vi "4Pi Capture Scan Counter.vi"(8 "Scan Tracker":T1) -> (0 "Scan Tracker Out":T1, 1 "Move stage?":bool, 2 "F_MVR/T_MOV":bool, 3 "Exit?":bool)   [LabVIEW 2021]
uses:
  4Pi Capture Manager Controls/4Pi Capture Scan Tracker.ctl
  4Pi Capture Manager Controls/4Pi Capture Switch Laser.ctl
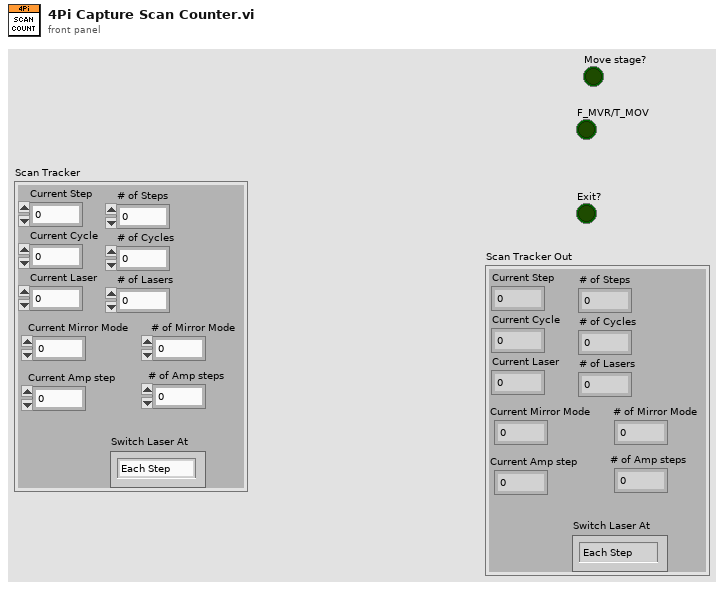
[diagram p1: front panel]
types:
  T1 = typedef "4Pi Capture Scan Tracker.ctl" = cluster{"Current Step":u16, "Current Cycle":u16, "Current Laser":u16, "# of Lasers":u16, "# of Cycles":u16, "# of Steps":u16, "Switch Laser At":T2, "Current Mirror Mode":u16, "# of Mirror Mode":u16, "Current Amp step":u16, "# of Amp steps":u16}
  T2 = typedef "4Pi Capture Switch Laser.ctl" = enum16{"Each Step", "Each Cycle", "All Cycles"}
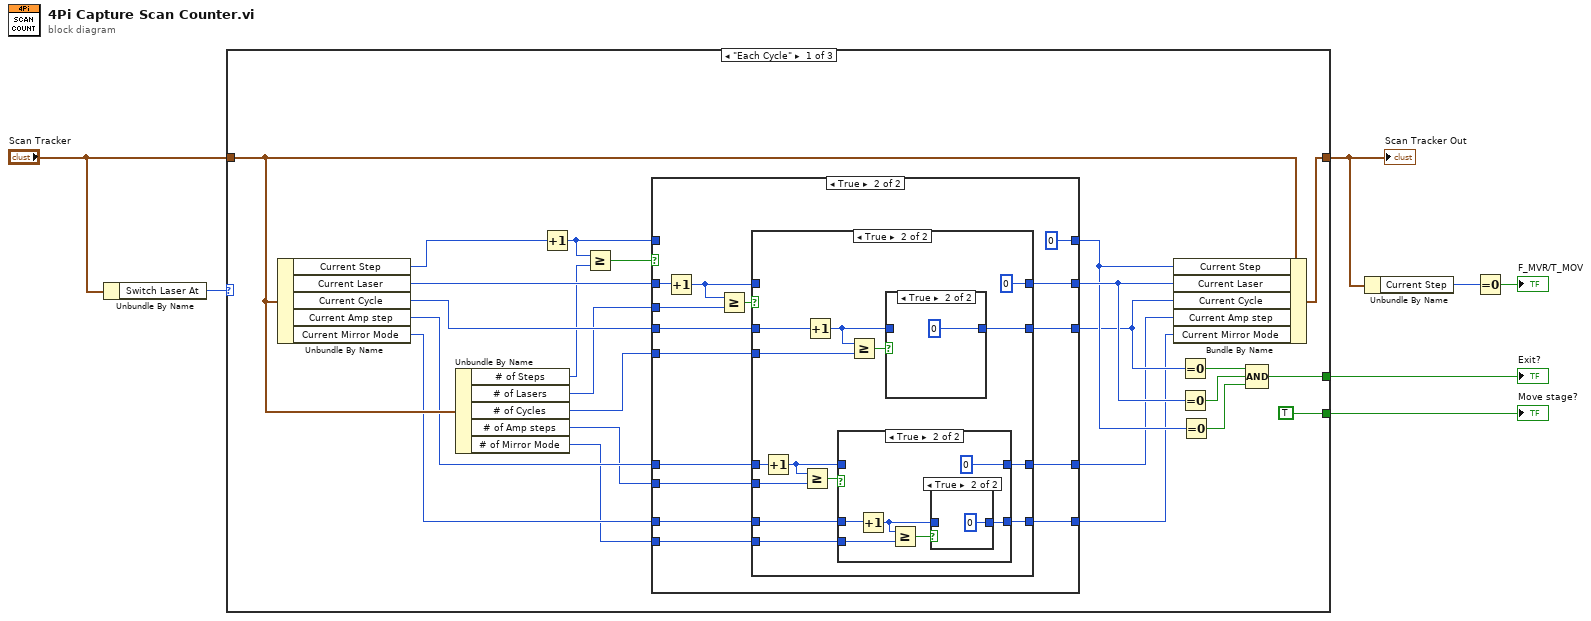
[diagram p0: block diagram]
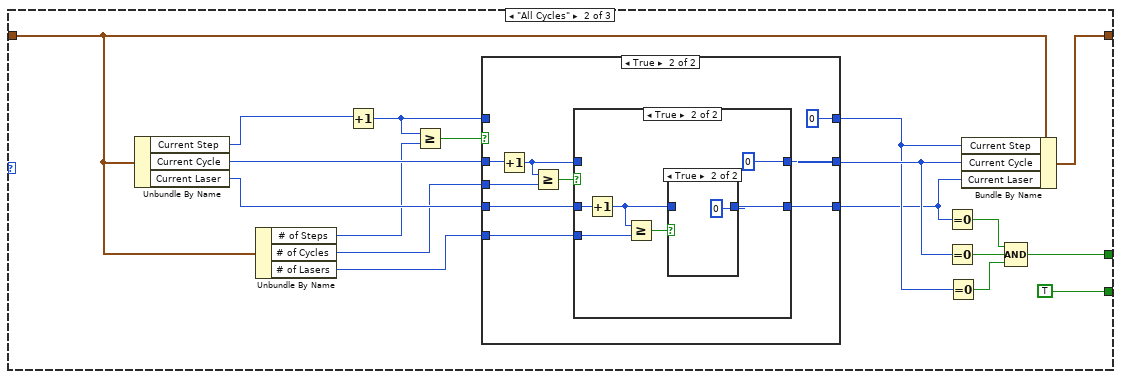
[diagram p7: hidden frame]
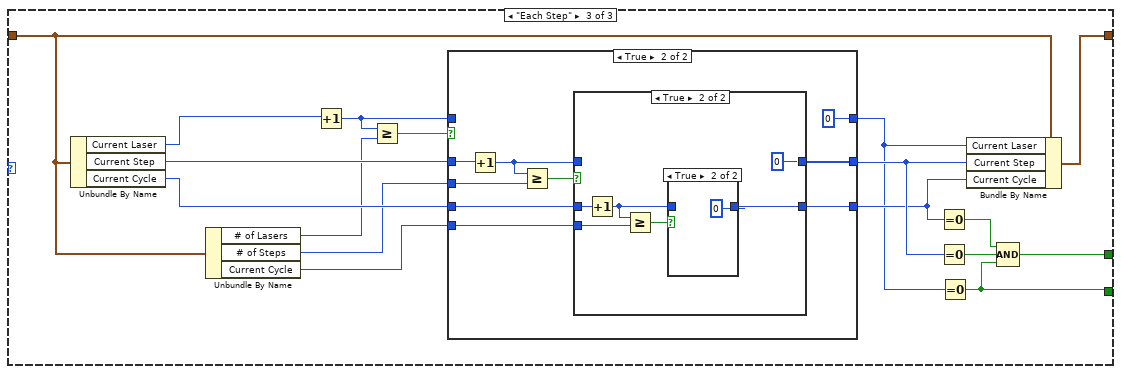
[diagram p11: hidden frame]
diagram:
  n1 = Unbundle By Name("Scan Tracker") -> ("Switch Laser At"=w7:T2)
  n2 = case shown="\"Each Cycle\"" w7 {
    tunnel: "Scan Tracker" -> [w15 w82 w122]
    tunnel: [w20 w87 w129] -> w3
    tunnel: [w19 w86 w128] -> w6
    tunnel: [TRUE TRUE w123] -> w2
    frame "Each Cycle" {
      n3 = Unbundle By Name(w15) -> ("Current Step"=w14:u16, "Current Laser"=w31:u16, "Current Cycle"=w30:u16, "Current Amp step"=w13:u16, "Current Mirror Mode"=w10:u16)
      n4 = Unbundle By Name(w15) -> ("# of Steps"=w17:u16, "# of Lasers"=w28:u16, "# of Cycles"=w27:u16, "# of Amp steps"=w12:u16, "# of Mirror Mode"=w9:u16)
      n5 = Increment(x=w14) -> (x+1=w18:u16)
      n6 = Greater Or Equal?(x=w18, y=w17) -> (x >= y?=w29:bool)
      n7 = case shown="True" w29 {
        tunnel: [w36 u16 0] -> w25
        tunnel: w18 -> [w36 _]
        tunnel: w31 -> [w35 w51]
        tunnel: w30 -> [w34 w46]
        tunnel: w28 -> [_ w43]
        tunnel: [w35 w48] -> w26
        tunnel: w27 -> [_ w47]
        tunnel: [w34 w45] -> w24
        tunnel: w13 -> [w33 w42]
        tunnel: w12 -> [_ w41]
        tunnel: [w33 w40] -> w11
        tunnel: w10 -> [w32 w39]
        tunnel: [w32 w38] -> w8
        tunnel: w9 -> [_ w37]
        frame False {
        }
        frame True {
          n8 = Increment(x=w51) -> (x+1=w44:u16)
          n9 = Greater Or Equal?(x=w44, y=w43) -> (x >= y?=w50:bool)
          n10 = case shown="True" w50 {
            tunnel: [w55 u16 0] -> w48
            tunnel: w44 -> [w55 _]
            tunnel: w47 -> [_ w64]
            tunnel: w46 -> [w54 w68]
            tunnel: [w54 w67] -> w45
            tunnel: w42 -> [w53 w63]
            tunnel: w41 -> [_ w62]
            tunnel: [w53 w59] -> w40
            tunnel: w39 -> [w52 w58]
            tunnel: [w52 w57] -> w38
            tunnel: w37 -> [_ w56]
            frame False {
            }
            frame True {
              n11 = Increment(x=w63) -> (x+1=w60:u16)
              n12 = Greater Or Equal?(x=w60, y=w62) -> (x >= y?=w61:bool)
              n13 = Increment(x=w68) -> (x+1=w65:u16)
              n14 = case shown="True" w61 {
                tunnel: w60 -> [w71 _]
                tunnel: [w71 u16 0] -> w59
                tunnel: w58 -> [w70 w76]
                tunnel: [w70 w72] -> w57
                tunnel: w56 -> [_ w75]
                frame False {
                }
                frame True {
                  n15 = Increment(x=w76) -> (x+1=w73:u16)
                  n16 = Greater Or Equal?(x=w73, y=w75) -> (x >= y?=w74:bool)
                  n17 = case shown="True" w74 {
                    tunnel: w73 -> [w78 _]
                    tunnel: [w78 u16 0] -> w72
                    frame False {
                    }
                    frame True {
                    }
                  }
                }
              }
              n18 = Greater Or Equal?(x=w65, y=w64) -> (x >= y?=w69:bool)
              n19 = case shown="True" w69 {
                tunnel: [w80 u16 0] -> w67
                tunnel: w65 -> [w80 _]
                frame False {
                }
                frame True {
                }
              }
            }
          }
        }
      }
      n20 = Bundle By Name(cluster=w15, "Current Step"=w25, "Current Laser"=w26, "Current Cycle"=w24, "Current Amp step"=w11, "Current Mirror Mode"=w8) -> (w19:T1)
      n21 = Equal To 0?(x=w24) -> (x = 0?=w23:bool)
      n22 = Equal To 0?(x=w26) -> (x = 0?=w22:bool)
      n23 = Equal To 0?(x=w25) -> (x = 0?=w21:bool)
      n24 = Compound Arithmetic op=AND(w23, w22, w21) -> (w20:bool)
    }
    frame "All Cycles" {
      n25 = Unbundle By Name(w82) -> ("Current Step"=w99:u16, "Current Cycle"=w98:u16, "Current Laser"=w97:u16)
      n26 = Unbundle By Name(w82) -> ("# of Steps"=w84:u16, "# of Cycles"=w95:u16, "# of Lasers"=w94:u16)
      n27 = Increment(x=w99) -> (x+1=w85:u16)
      n28 = Greater Or Equal?(x=w85, y=w84) -> (x >= y?=w96:bool)
      n29 = case shown="True" w96 {
        tunnel: [w102 u16 0] -> w92
        tunnel: w85 -> [w102 _]
        tunnel: w98 -> [w101 w111]
        tunnel: w97 -> [w100 w106]
        tunnel: w95 -> [_ w104]
        tunnel: [w101 w108] -> w93
        tunnel: w94 -> [_ w107]
        tunnel: [w100 w105] -> w91
        frame False {
        }
        frame True {
          n30 = Increment(x=w111) -> (x+1=w103:u16)
          n31 = Greater Or Equal?(x=w103, y=w104) -> (x >= y?=w110:bool)
          n32 = case shown="True" w110 {
            tunnel: [w113 u16 0] -> w108
            tunnel: w103 -> [w113 _]
            tunnel: w107 -> [_ w115]
            tunnel: w106 -> [w112 w118]
            tunnel: [w112 w117] -> w105
            frame False {
            }
            frame True {
              n33 = Increment(x=w118) -> (x+1=w114:u16)
              n34 = Greater Or Equal?(x=w114, y=w115) -> (x >= y?=w119:bool)
              n35 = case shown="True" w119 {
                tunnel: [w120 u16 0] -> w117
                tunnel: w114 -> [w120 _]
                frame False {
                }
                frame True {
                }
              }
            }
          }
        }
      }
      n36 = Equal To 0?(x=w91) -> (x = 0?=w90:bool)
      n37 = Equal To 0?(x=w93) -> (x = 0?=w89:bool)
      n38 = Equal To 0?(x=w92) -> (x = 0?=w88:bool)
      n39 = Bundle By Name(cluster=w82, "Current Step"=w92, "Current Cycle"=w93, "Current Laser"=w91) -> (w86:T1)
      n40 = Compound Arithmetic op=AND(w90, w89, w88) -> (w87:bool)
    }
    frame "Each Step" {
      n41 = Unbundle By Name(w122) -> ("Current Laser"=w138:u16, "Current Step"=w137:u16, "Current Cycle"=w136:u16)
      n42 = Unbundle By Name(w122) -> ("# of Lasers"=w126:u16, "# of Steps"=w125:u16, "Current Cycle"=w134:u16)
      n43 = Increment(x=w138) -> (x+1=w127:u16)
      n44 = Greater Or Equal?(x=w127, y=w126) -> (x >= y?=w135:bool)
      n45 = case shown="True" w135 {
        tunnel: [w141 u16 0] -> w124
        tunnel: w127 -> [w141 _]
        tunnel: w137 -> [w140 w150]
        tunnel: w136 -> [w139 w145]
        tunnel: w125 -> [_ w142]
        tunnel: [w140 w147] -> w133
        tunnel: w134 -> [_ w146]
        tunnel: [w139 w144] -> w132
        frame False {
        }
        frame True {
          n46 = Increment(x=w150) -> (x+1=w143:u16)
          n47 = Greater Or Equal?(x=w143, y=w142) -> (x >= y?=w149:bool)
          n48 = case shown="True" w149 {
            tunnel: [w152 u16 0] -> w147
            tunnel: w143 -> [w152 _]
            tunnel: w146 -> [_ w153]
            tunnel: w145 -> [w151 w157]
            tunnel: [w151 w156] -> w144
            frame False {
            }
            frame True {
              n49 = Increment(x=w157) -> (x+1=w154:u16)
              n50 = Greater Or Equal?(x=w154, y=w153) -> (x >= y?=w158:bool)
              n51 = case shown="True" w158 {
                tunnel: [w159 u16 0] -> w156
                tunnel: w154 -> [w159 _]
                frame False {
                }
                frame True {
                }
              }
            }
          }
        }
      }
      n52 = Equal To 0?(x=w132) -> (x = 0?=w131:bool)
      n53 = Equal To 0?(x=w133) -> (x = 0?=w130:bool)
      n54 = Equal To 0?(x=w124) -> (x = 0?=w123:bool)
      n55 = Bundle By Name(cluster=w122, "Current Laser"=w124, "Current Step"=w133, "Current Cycle"=w132) -> (w128:T1)
      n56 = Compound Arithmetic op=AND(w131, w130, w123) -> (w129:bool)
    }
  }
  "Exit?" <- w3
  "Move stage?" <- w2
  "Scan Tracker Out" <- w6
  n57 = Unbundle By Name(w6) -> ("Current Step"=w5:u16)
  n58 = Equal To 0?(x=w5) -> (x = 0?=→"F_MVR/T_MOV":bool)
